vi "_Remove Variable Source File in Map.vi"(7 "String":string, 8 "error in (no error)":errorcluster, 9 "dup path":path, 10 "Content":string, 11 "Variable-FileMap":variant) -> (0 "error out":errorcluster, 1 "No Source Any More?":bool, 2 "Latest File Path (If changed)":path, 3 "Variant":variant)   [LabVIEW 2017, in "INI-Static-Variable-Support.lvlib" / "CSM-Static-Variable-Manager.lvclass"]
uses:
  CSM-Static-Variable-Manager.lvclass
  <userlib>/_NEVSTOP/Communicable State Machine(CSM)/addons/API-String-Arugments-Support/API String Arguments Support.lvlib
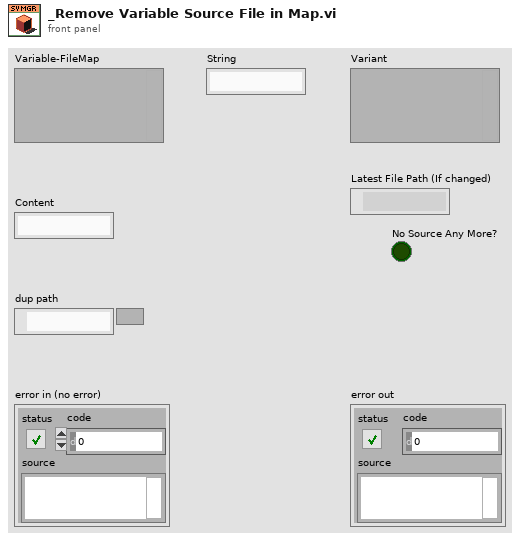
[diagram p1: front panel]
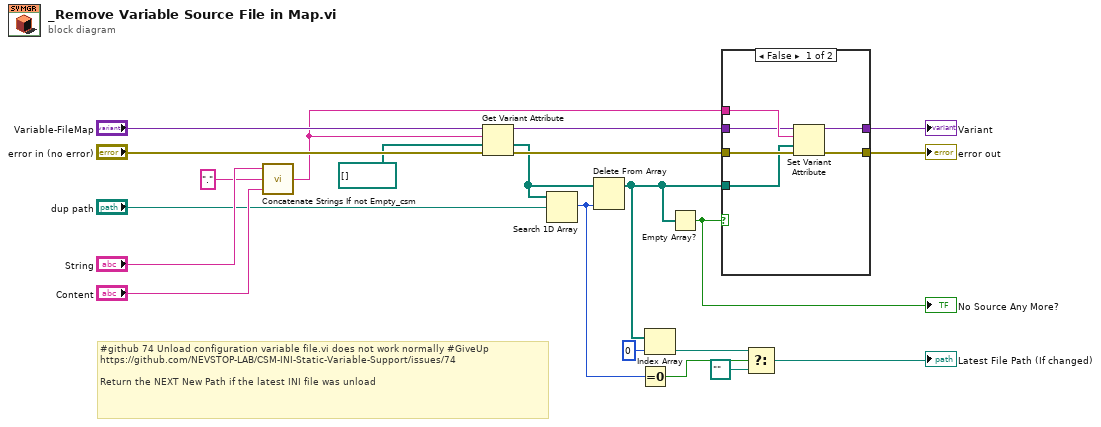
[diagram p0: block diagram]
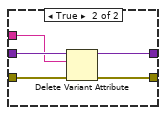
[diagram p2: hidden frame]
diagram:
  # "#github 74 Unload configuration variable file.vi does not work normally #GiveUp\nhttps://github.com/NEVSTOP-LAB/CSM-INI-Static-Variable-Support/issues/74\n\nReturn the NEXT New Path if the latest INI file was unload"
  n1 = call <userlib>:"Concatenate Strings If not Empty_csm.vi"("String"="Content", "seperator(:)"=".", "prefix"="String") -> ("result"=w16:string)  [unwired: 2 in]
  n2 = Get Variant Attribute(Variant="Variable-FileMap", name=w16, default value (empty Variant)=path[] [], error in="error in (no error)") -> (duplicate Variant=w15:variant, value=w9:path[], error out=w17:errorcluster)  [unwired: 1 out]
  n3 = Search 1D Array(1D array=w9, element="dup path") -> (index of element=w6:i32)  [unwired: 1 in]
  n4 = Delete From Array(array=w9, index=w6) -> (array with subset deleted=w4:path[])  [unwired: 1 in, 1 out]
  n5 = Equal To 0?(x=w6) -> (x = 0?=w7:bool)
  n6 = Index Array(array=w4, index=0) -> (element=w5:path)
  n7 = Empty Array?(array=w4) -> (empty?=w8:bool)
  "No Source Any More?" <- w8
  n8 = case shown="False" w8 {
    tunnel: [w27 w29] -> w21
    tunnel: [w26 w31] -> w19
    tunnel: w17 -> [w25 w30]
    tunnel: w16 -> [w24 w28]
    tunnel: w15 -> [w23 w32]
    tunnel: w4 -> [w22 _]
    frame False {
      n9 = Set Variant Attribute(Variant=w23, name=w24, value=w22, error in=w25) -> (Variant out=w26:variant, error out=w27:errorcluster)  [unwired: 1 out]
    }
    frame True {
      n10 = Delete Variant Attribute(4:w30, 6:w28, 7:w32) -> (0:w29:errorcluster, 3:w31:variant)  [unwired: 1 out]
    }
  }
  "error out" <- w21
  "Variant" <- w19
  n11 = Select(t=w5, s=w7, f=path "") -> (s? t:f=→"Latest File Path (If changed)":path)
